vi "Init.vi"(8 "error in (no error)":errorcluster, 9 "Frequencies":dbl[](array[numeric]), 10 "SA Pin":string, 11 "Measurement Name":string) -> (0 "error out":errorcluster, 3 "Skyworks_SpurTest out":refnum<class "Skyworks_SpurTest.lvclass">)   [LabVIEW 2016, in "SeqAuto Evaluations.lvlib" / "Skyworks_SpurTest.lvclass"]
uses:
  Skyworks_SpurTest.lvclass
  C:/Sequence Automation/Plugins/SeqAuto IEvaluation.lvlibp/SeqAuto IEvaluation.lvclass
  Skyworks_SpurTest.lvclass/Skyworks_SpurTest.ctl
  Plugins/SeqAuto IEvaluation.lvlibp/Write Measurement Name.vi
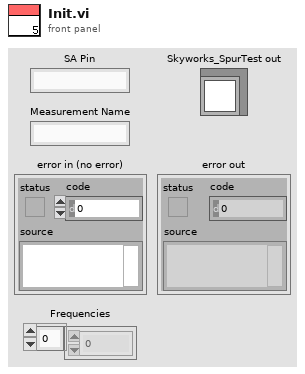
[diagram p1: front panel]
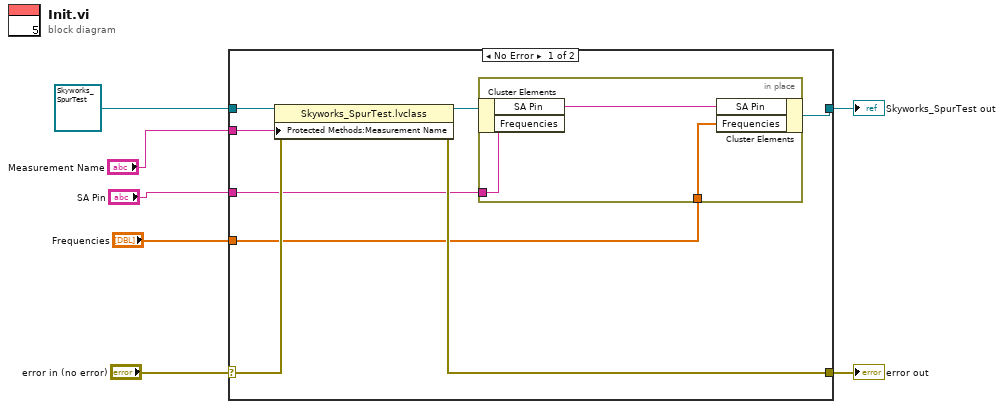
[diagram p0: block diagram]
diagram:
  n1 = case shown="No Error" "error in (no error)" {
    selector: "error in (no error)" -> [w15 w19]
    tunnel: [w14 w19] -> w6
    tunnel: [w9 w18] -> w5
    tunnel: refnum<class "Skyworks_SpurTest.lvclass"> refnum ("Skyworks_SpurTest in") -> [w13 w18]
    tunnel: "Measurement Name" -> [w11 _]
    tunnel: "SA Pin" -> [w10 _]
    tunnel: "Frequencies" -> [w8 _]
    frame No Error {
      n2 = property class="Skyworks_SpurTest.lvclass"(reference=w13, error in=w15, "Protected Methods:Measurement Name"=w11) -> (reference out=w12:refnum<class "Skyworks_SpurTest.lvclass">, error out=w14:errorcluster)
      n3 = in-place {
        in-place-border: w10 -> [w17]
        in-place-border: w8 -> [w16]
        n4 = in-place-cluster #1(w12) -> ()  [unwired: 2 out]
        n5 = in-place-cluster #1("SA Pin"=w17, "Frequencies"=w16) -> (w9:refnum<class "Skyworks_SpurTest.lvclass">)
      }
    }
    frame Error {
    }
  }
  "error out" <- w6
  "Skyworks_SpurTest out" <- w5
